vi "Add Component Default Settings.vi"(8 "error in (no error)":errorcluster, 10 "Component":refnum<class "Component.lvclass">, 11 "framework configuration in":T1) -> (0 "error out":errorcluster, 3 "framework configuration out":T1)   [LabVIEW 2019, in "DSF Core.lvlib"]
uses:
  DSF Core.lvlib
  Typedefs/DSF Engine Framework Configuration.ctl
  Typedefs/DSF Engine Plugin Configuration.ctl
  Typedefs/Core Plugin Configuration.ctl
  Typedefs/DSF Timing Info.ctl
  Typedefs/DSF Settings Info.ctl
  Typedefs/DSF Engine Plugin Thread Configuration.ctl
  Typedefs/Core Thread Configuration.ctl
  Typedefs/DSF Engine Transfer Group Configuration.ctl
  Typedefs/Core Group Configuration.ctl
  Typedefs/DSF Direction.ctl
  Typedefs/DSF Timeout Behavior.ctl
  Typedefs/DSF Engine Transfer Configuration.ctl
  Typedefs/Core Transfer Configuration.ctl
  Typedefs/DSF Engine Channel Configuration.ctl
  Typedefs/Core Channel Configuration.ctl
  Typedefs/DSF Data Type.ctl
  Classes/Component/Component.lvclass
  Classes/Component/Component.lvclass/Component.ctl
  Classes/Component Configuration/Component Configurations.lvclass
  Classes/Configuration/Configuration.lvclass
  Classes/Configuration/Core/Plugin/Plugin Configuration.lvclass
  Classes/Configuration/Core/Thread/Thread Configuration.lvclass
  Classes/Configuration/Core/Group/Group Configuration.lvclass
  Classes/Configuration/Core/Transfer/Transfer Configuration.lvclass
  Classes/Configuration/Core/Channel/Channel Configuration.lvclass
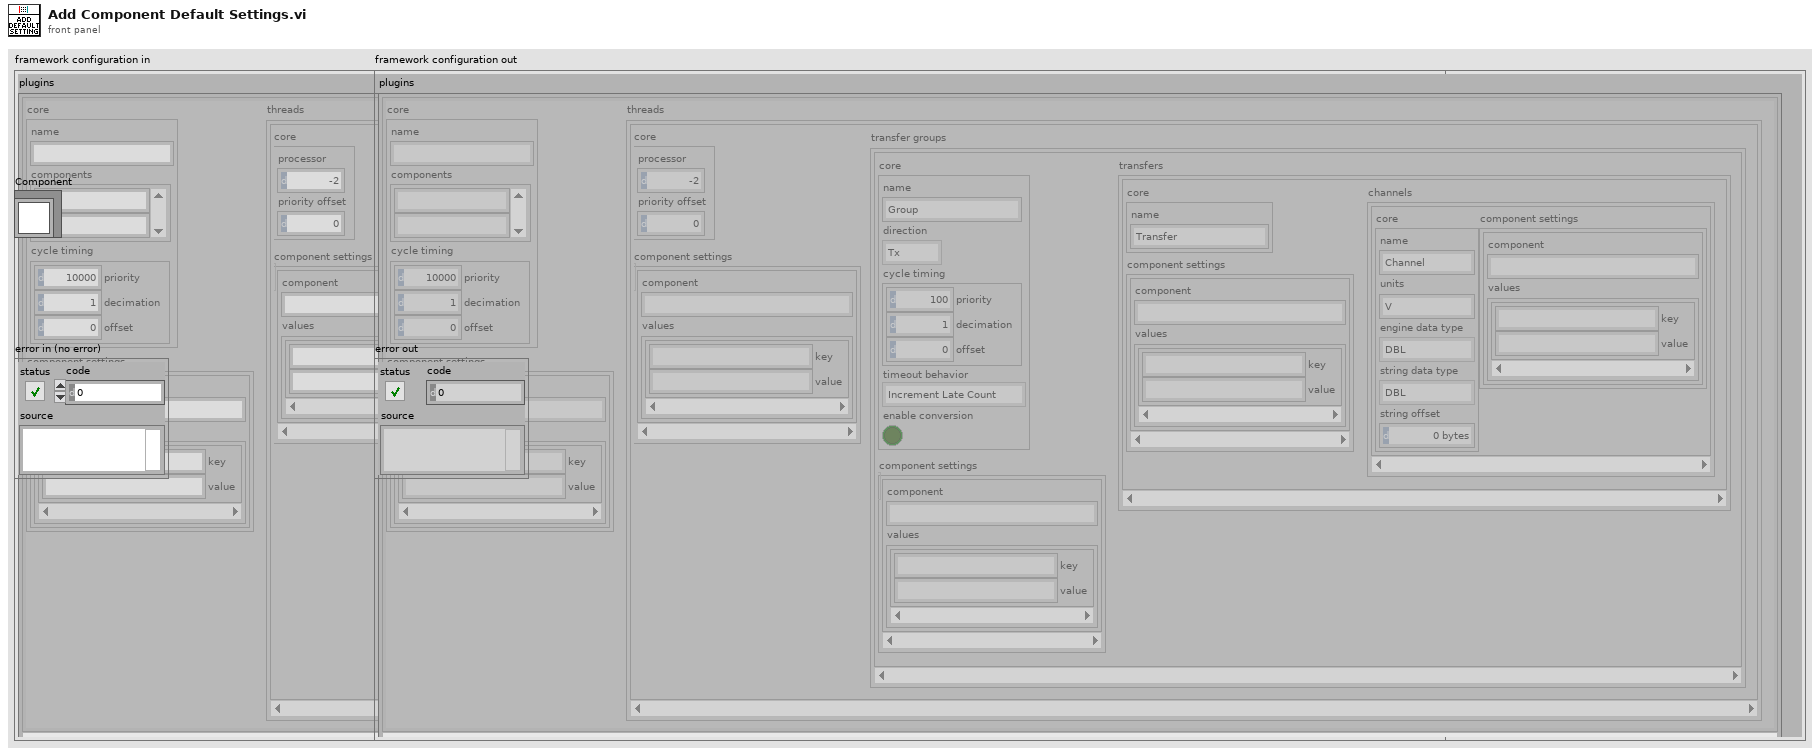
[diagram p1: front panel]
types:
  T1 = typedef "DSF Core.lvlib/DSF Engine Framework Configuration.ctl" = cluster{"plugins":T2[]}
  T2 = typedef "DSF Core.lvlib/DSF Engine Plugin Configuration.ctl" = cluster{"core":T3, "component settings":T5[], "threads":T6[]}
  T3 = typedef "DSF Core.lvlib/Plugin Configuration.lvclass/Core Plugin Configuration.ctl" = cluster{"name":string, "components":string[], "cycle timing":T4}
  T4 = typedef "DSF Core.lvlib/DSF Timing Info.ctl" = cluster{"priority":u64, "decimation":u64, "offset":u64}
  T5 = typedef "DSF Core.lvlib/DSF Settings Info.ctl" = cluster{"component":string, "values":cluster{"key":string, "value":string}[]}
  T6 = typedef "DSF Core.lvlib/DSF Engine Plugin Thread Configuration.ctl" = cluster{"core":T7, "component settings":T5[], "transfer groups":T8[]}
  T7 = typedef "DSF Core.lvlib/Thread Configuration.lvclass/Core Thread Configuration.ctl" = cluster{"processor":i32, "priority offset":i16}
  T8 = typedef "DSF Core.lvlib/DSF Engine Transfer Group Configuration.ctl" = cluster{"core":T9, "component settings":T5[], "transfers":T12[]}
  T9 = typedef "DSF Core.lvlib/Group Configuration.lvclass/Core Group Configuration.ctl" = cluster{"name":string, "direction":T10, "cycle timing":T4, "timeout behavior":T11, "enable conversion":bool}
  T10 = typedef "DSF Core.lvlib/DSF Direction.ctl" = enum8{"Tx", "Rx"}
  T11 = typedef "DSF Core.lvlib/DSF Timeout Behavior.ctl" = enum8{"Increment Late Count", "Throw Error"}
  T12 = typedef "DSF Core.lvlib/DSF Engine Transfer Configuration.ctl" = cluster{"core":T13, "component settings":T5[], "channels":T14[]}
  T13 = typedef "DSF Core.lvlib/Transfer Configuration.lvclass/Core Transfer Configuration.ctl" = cluster{"name":string}
  T14 = typedef "DSF Core.lvlib/DSF Engine Channel Configuration.ctl" = cluster{"core":T15, "component settings":T5[]}
  T15 = typedef "DSF Core.lvlib/Channel Configuration.lvclass/Core Channel Configuration.ctl" = cluster{"name":string, "units":string, "engine data type":T16, "string data type":T16, "string offset":u64}
  T16 = typedef "DSF Core.lvlib/DSF Data Type.ctl" = enum8{"Bool", "SGL", "DBL", "I8", "I16", "I32", "I64", "U8", "U16", "U32", "U64"}
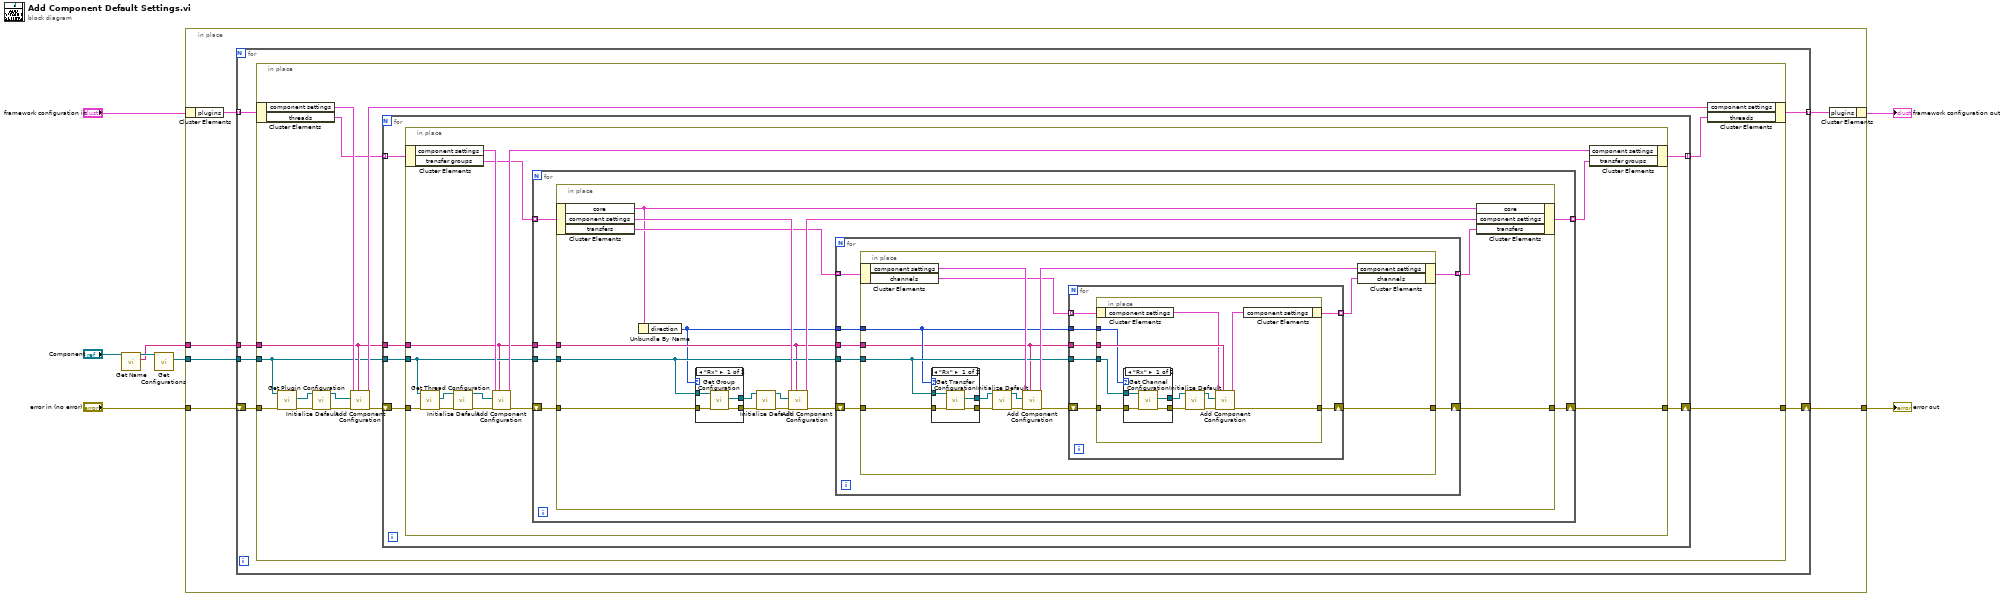
[diagram p0: block diagram]
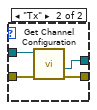
[diagram p2: hidden frame]
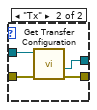
[diagram p3: hidden frame]
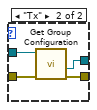
[diagram p4: hidden frame]
diagram:
  n1 = call "Get Name.vi"("Component in"="Component") -> ("name"=w3:string, "Component out"=w5:refnum<class "Component.lvclass">)  [unwired: 9 in]
  n2 = call "Get Configurations.vi"("Component in"=w5) -> ("Configurations"=w4:refnum<class "Component Configurations.lvclass">)  [unwired: 9 in, 1 out]
  n3 = in-place {
    in-place-border: w4 -> [w12]
    in-place-border: w3 -> [w11]
    in-place-border: "error in (no error)" -> [w10]
    in-place-border: [w9] -> w1
    n4 = in-place-cluster #1("framework configuration in") -> ("plugins"=w14:T2[])
    n5 = for {
      tunnel: w14 -> [w19] mode=indexing
      tunnel: [w20] -> w13 mode=indexing
      tunnel: w12 -> [w18]
      tunnel: w11 -> [w17]
      shift-right: [w15] -> w9
      shift-left: w10 -> [w16]
      n6 = in-place {
        in-place-border: w18 -> [w22]
        in-place-border: w17 -> [w24]
        in-place-border: w16 -> [w27]
        in-place-border: [w21] -> w15
        n7 = in-place-cluster #2(w19) -> ("component settings"=w29:T5[], "threads"=w26:T6[])
        n8 = call-dynamic "Get Plugin Configuration.vi"("error in (no error)"=w27, "Component Configuration in"=w22) -> ("error out"=w32:errorcluster, "Plugin Configuration"=w33:refnum<class "Configuration.lvclass">)  [unwired: 7 in, 1 out]
        n9 = call-dynamic "Initialize Default.vi"("error in (no error)"=w32, "Configuration in"=w33) -> ("error out"=w28:errorcluster, "Configuration out"=w31:refnum<class "Configuration.lvclass">)  [unwired: 8 in]
        n10 = call "Add Component Configuration.vi"("component name"=w24, "error in (no error)"=w28, "Configuration"=w31, "component settings in"=w29) -> ("error out"=w23:errorcluster, "component settings out"=w30:T5[])  [unwired: 5 in, 1 out]
        n11 = for {
          tunnel: w26 -> [w39] mode=indexing
          tunnel: [w38] -> w25 mode=indexing
          tunnel: w24 -> [w37]
          shift-right: [w34] -> w21
          shift-left: w23 -> [w36]
          tunnel: w22 -> [w35]
          n12 = in-place {
            in-place-border: w37 -> [w43]
            in-place-border: w36 -> [w48]
            in-place-border: w35 -> [w44]
            in-place-border: [w41] -> w34
            n13 = in-place-cluster #3(w39) -> ("component settings"=w50:T5[], "transfer groups"=w45:T8[])
            n14 = call-dynamic "Get Thread Configuration.vi"("error in (no error)"=w48, "Component Configuration in"=w44) -> ("error out"=w47:errorcluster, "Thread Configuration"=w46:refnum<class "Configuration.lvclass">)  [unwired: 7 in, 1 out]
            n15 = call-dynamic "Initialize Default.vi"("error in (no error)"=w47, "Configuration in"=w46) -> ("error out"=w51:errorcluster, "Configuration out"=w52:refnum<class "Configuration.lvclass">)  [unwired: 8 in]
            n16 = call "Add Component Configuration.vi"("component name"=w43, "error in (no error)"=w51, "Configuration"=w52, "component settings in"=w50) -> ("error out"=w42:errorcluster, "component settings out"=w49:T5[])  [unwired: 5 in, 1 out]
            n17 = for {
              tunnel: w45 -> [w58] mode=indexing
              tunnel: w44 -> [w57]
              tunnel: w43 -> [w56]
              shift-right: [w54] -> w41
              shift-left: w42 -> [w55]
              tunnel: [w53] -> w40 mode=indexing
              n18 = in-place {
                in-place-border: w57 -> [w64]
                in-place-border: w56 -> [w63]
                in-place-border: w55 -> [w73]
                in-place-border: [w61] -> w54
                n19 = in-place-cluster #4(w58) -> ("core"=w59:T9, "component settings"=w69:T5[], "transfers"=w66:T12[])
                n20 = Unbundle By Name(w59) -> ("direction"=w62:T10)
                n21 = case shown="\"Rx\"" w62 {
                  tunnel: w64 -> [w131 w135]
                  tunnel: w73 -> [w132 w136]
                  tunnel: [w130 w134] -> w72
                  tunnel: [w129 w133] -> w71
                  frame "Rx" {
                    n22 = call-dynamic "Get Group Configuration.vi"("error in (no error)"=w132, "Component Configuration in"=w131) -> ("error out"=w130:errorcluster, "Rx Group Configuration"=w129:refnum<class "Configuration.lvclass">)  [unwired: 6 in, 2 out]
                  }
                  frame "Tx" {
                    n23 = call-dynamic "Get Group Configuration.vi"("error in (no error)"=w136, "Component Configuration in"=w135) -> ("error out"=w134:errorcluster, "Tx Group Configuration"=w133:refnum<class "Configuration.lvclass">)  [unwired: 6 in, 2 out]
                  }
                }
                n24 = call-dynamic "Initialize Default.vi"("error in (no error)"=w72, "Configuration in"=w71) -> ("error out"=w70:errorcluster, "Configuration out"=w67:refnum<class "Configuration.lvclass">)  [unwired: 8 in]
                n25 = call "Add Component Configuration.vi"("component name"=w63, "error in (no error)"=w70, "Configuration"=w67, "component settings in"=w69) -> ("error out"=w65:errorcluster, "component settings out"=w68:T5[])  [unwired: 5 in, 1 out]
                n26 = for {
                  tunnel: w66 -> [w80] mode=indexing
                  tunnel: w62 -> [w79]
                  shift-right: [w75] -> w61
                  shift-left: w65 -> [w78]
                  tunnel: w64 -> [w77]
                  tunnel: w63 -> [w76]
                  tunnel: [w74] -> w60 mode=indexing
                  n27 = in-place {
                    in-place-border: w79 -> [w84]
                    in-place-border: w78 -> [w90]
                    in-place-border: w77 -> [w85]
                    in-place-border: w76 -> [w83]
                    in-place-border: [w82] -> w75
                    n28 = in-place-cluster #5(w80) -> ("component settings"=w89:T5[], "channels"=w87:T14[])
                    n29 = case shown="\"Rx\"" w84 {
                      tunnel: w85 -> [w123 w127]
                      tunnel: w90 -> [w124 w128]
                      tunnel: [w122 w126] -> w94
                      tunnel: [w121 w125] -> w93
                      frame "Rx" {
                        n30 = call-dynamic "Get Transfer Configuration.vi"("error in (no error)"=w124, "Component Configuration in"=w123) -> ("error out"=w122:errorcluster, "Rx Transfer Configuration"=w121:refnum<class "Configuration.lvclass">)  [unwired: 6 in, 2 out]
                      }
                      frame "Tx" {
                        n31 = call-dynamic "Get Transfer Configuration.vi"("error in (no error)"=w128, "Component Configuration in"=w127) -> ("error out"=w126:errorcluster, "Tx Transfer Configuration"=w125:refnum<class "Configuration.lvclass">)  [unwired: 6 in, 2 out]
                      }
                    }
                    n32 = call-dynamic "Initialize Default.vi"("error in (no error)"=w94, "Configuration in"=w93) -> ("error out"=w92:errorcluster, "Configuration out"=w91:refnum<class "Configuration.lvclass">)  [unwired: 8 in]
                    n33 = call "Add Component Configuration.vi"("component name"=w83, "error in (no error)"=w92, "Configuration"=w91, "component settings in"=w89) -> ("error out"=w86:errorcluster, "component settings out"=w88:T5[])  [unwired: 5 in, 1 out]
                    n34 = for {
                      tunnel: w87 -> [w101] mode=indexing
                      shift-right: [w99] -> w82
                      shift-left: w86 -> [w100]
                      tunnel: w85 -> [w98]
                      tunnel: w84 -> [w96]
                      tunnel: w83 -> [w97]
                      tunnel: [w95] -> w81 mode=indexing
                      n35 = in-place {
                        in-place-border: w100 -> [w108]
                        in-place-border: [w107] -> w99
                        in-place-border: w98 -> [w106]
                        in-place-border: w97 -> [w105]
                        in-place-border: w96 -> [w104]
                        n36 = in-place-cluster #6(w101) -> ("component settings"=w103:T5[])
                        n37 = case shown="\"Rx\"" w104 {
                          tunnel: w106 -> [w115 w119]
                          tunnel: w108 -> [w116 w120]
                          tunnel: [w113 w118] -> w112
                          tunnel: [w114 w117] -> w111
                          frame "Rx" {
                            n38 = call-dynamic "Get Channel Configuration.vi"("error in (no error)"=w116, "Component Configuration in"=w115) -> ("error out"=w113:errorcluster, "Rx Channel Configuration"=w114:refnum<class "Configuration.lvclass">)  [unwired: 6 in, 2 out]
                          }
                          frame "Tx" {
                            n39 = call-dynamic "Get Channel Configuration.vi"("error in (no error)"=w120, "Component Configuration in"=w119) -> ("error out"=w118:errorcluster, "Tx Channel Configuration"=w117:refnum<class "Configuration.lvclass">)  [unwired: 6 in, 2 out]
                          }
                        }
                        n40 = call-dynamic "Initialize Default.vi"("error in (no error)"=w112, "Configuration in"=w111) -> ("error out"=w110:errorcluster, "Configuration out"=w109:refnum<class "Configuration.lvclass">)  [unwired: 8 in]
                        n41 = call "Add Component Configuration.vi"("component name"=w105, "error in (no error)"=w110, "Configuration"=w109, "component settings in"=w103) -> ("error out"=w107:errorcluster, "component settings out"=w102:T5[])  [unwired: 5 in, 1 out]
                        n42 = in-place-cluster #6("component settings"=w102) -> (w95:T14)
                      }
                    }
                    n43 = in-place-cluster #5("component settings"=w88, "channels"=w81) -> (w74:T12)
                  }
                }
                n44 = in-place-cluster #4("core"=w59, "component settings"=w68, "transfers"=w60) -> (w53:T8)
              }
            }
            n45 = in-place-cluster #3("component settings"=w49, "transfer groups"=w40) -> (w38:T6)
          }
        }
        n46 = in-place-cluster #2("component settings"=w30, "threads"=w25) -> (w20:T2)
      }
    }
    n47 = in-place-cluster #1("plugins"=w13) -> (→"framework configuration out":T1)
  }
  "error out" <- w1
